vi "SubVI_Write ini file.vi"(8 "Path":path=path "C:/labview project/PSA SubVIs/ini file/Spec An Settings.ini", 10 "Frequency Range":T1, 11 "Prescan Spec An Setting":T2={"Reference Level (dBuV)"=107.0, "Attenuation (dB)"=10.0, "Step Size (KHz)"=90.0, "RBW (KHz)"=120.0, "VBW (KHz)"=300.0, "Dwell Time (ms)"=0.1, "Detector"=enum."Peak"}) -> ()   [LabVIEW 2016]
doc: "create INI file for different frequency band in different program status"
uses:
  Prescan Spec An Setting.ctl
  Frequency Range.ctl
  <vilib>/Utility/config.llb/Write Key (String).vi
  <vilib>/Utility/config.llb/Write Key (Double).vi
  <vilib>/Utility/config.llb/NI_LVConfig.lvlib
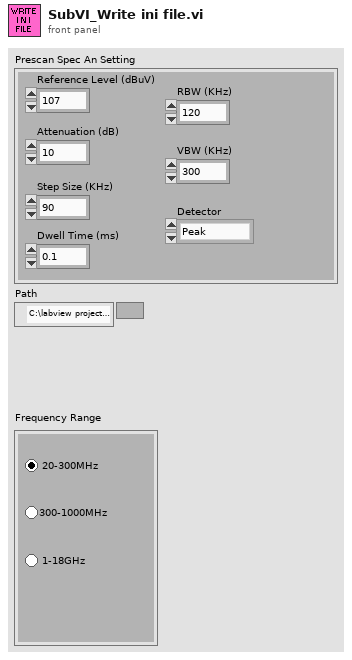
[diagram p1: front panel]
types:
  T1 = typedef "Frequency Range.ctl" = enum32{"20-300MHz", "300-1000MHz", "1-18GHz"}
  T2 = typedef "Prescan Spec An Setting.ctl" = cluster{"Reference Level (dBuV)":dbl, "Attenuation (dB)":dbl, "Step Size (KHz)":dbl, "RBW (KHz)":dbl, "VBW (KHz)":dbl, "Dwell Time (ms)":dbl, "Detector":enum16{"Peak", "CISPR Peak", "Mil Peak", "Quasi Peak", "Average"}}
  T3 = enum16{"Peak", "CISPR Peak", "Mil Peak", "Quasi Peak", "Average"}
  T4 = typedef "NI_LVConfig.lvlib/Config Data RefNum.ctl" = refnum<k1>
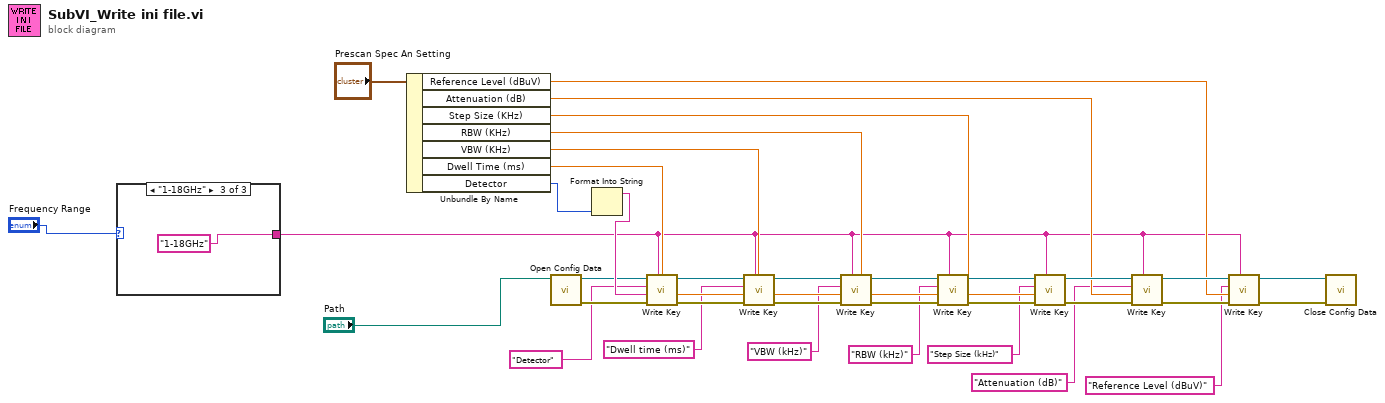
[diagram p0: block diagram]
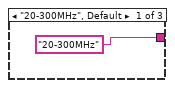
[diagram p2: hidden frame]
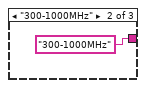
[diagram p3: hidden frame]
diagram:
  n1 = case shown="\"1-18GHz\"" "Frequency Range" {
    tunnel: ["20-300MHz" "300-1000MHz" "1-18GHz"] -> w1
    frame "20-300MHz", Default {
    }
    frame "300-1000MHz" {
    }
    frame "1-18GHz" {
    }
  }
  n2 = Unbundle By Name("Prescan Spec An Setting") -> ("Reference Level (dBuV)"=w18:dbl, "Attenuation (dB)"=w19:dbl, "Step Size (KHz)"=w20:dbl, "RBW (KHz)"=w21:dbl, "VBW (KHz)"=w22:dbl, "Dwell Time (ms)"=w23:dbl, "Detector"=w15:T3)
  n3 = call <vilib>:"Open Config Data.vi"("configuration file path"="Path") -> ("error out"=w12:errorcluster, "refnum"=w13:T4)  [unwired: 8 in, 1 out]
  n4 = Format Into String(w15) -> (resulting string=w14:string)  [unwired: 3 in, 1 out]
  n5 = call-poly <vilib>:"Write Key.vi"("section"=w1, "error in (no error)"=w12, "value"=w14, "key"="Detector", "refnum"=w13) -> ("error out"=w9:errorcluster, "refnum out"=w10:T4)  [unwired: 4 in, 1 out]
  n6 = call-poly <vilib>:"Write Key.vi"("section"=w1, "error in (no error)"=w9, "value"=w23, "key"="Dwell time (ms)", "refnum"=w10) -> ("error out"=w34:errorcluster, "refnum out"=w33:T4)  [unwired: 4 in, 1 out]
  n7 = call-poly <vilib>:"Write Key.vi"("section"=w1, "error in (no error)"=w34, "value"=w22, "key"="VBW (kHz)", "refnum"=w33) -> ("error out"=w30:errorcluster, "refnum out"=w29:T4)  [unwired: 4 in, 1 out]
  n8 = call-poly <vilib>:"Write Key.vi"("section"=w1, "error in (no error)"=w30, "value"=w21, "key"="RBW (kHz)", "refnum"=w29) -> ("error out"=w31:errorcluster, "refnum out"=w32:T4)  [unwired: 4 in, 1 out]
  n9 = call-poly <vilib>:"Write Key.vi"("section"=w1, "error in (no error)"=w31, "value"=w20, "key"="Step Size (kHz)", "refnum"=w32) -> ("error out"=w26:errorcluster, "refnum out"=w25:T4)  [unwired: 4 in, 1 out]
  n10 = call-poly <vilib>:"Write Key.vi"("section"=w1, "error in (no error)"=w26, "value"=w19, "key"="Attenuation (dB)", "refnum"=w25) -> ("error out"=w27:errorcluster, "refnum out"=w28:T4)  [unwired: 4 in, 1 out]
  n11 = call-poly <vilib>:"Write Key.vi"("section"=w1, "error in (no error)"=w27, "value"=w18, "key"="Reference Level (dBuV)", "refnum"=w28) -> ("error out"=w16:errorcluster, "refnum out"=w17:T4)  [unwired: 4 in, 1 out]
  n12 = call <vilib>:"Close Config Data.vi"("error in (no error)"=w16, "refnum"=w17) -> ()  [unwired: 8 in, 2 out]
